vi "GetPos.vi"(0 "Axis In":T1=enum."Y", 11 "error in (no error)":errorcluster) -> (4 "Axis Out":T1=enum."Y", 6 "Position":dbl, 10 "Encoder Counts":i32, 15 "error out":errorcluster)   [LabVIEW 2009]
uses:
  typedefs/AxisSelect_Enum.ctl
  globals/AxisSpace.vi
  typedefs/Ultra3000/Func.ctl
  typedefs/Ultra3000/Cmds.ctl
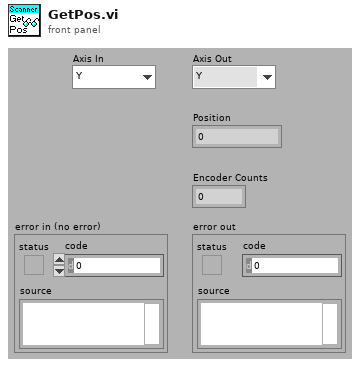
[diagram p1: front panel]
types:
  T1 = typedef "AxisSelect_Enum.ctl" = enum16{"X", "Y", "Z", "Axis Space"}
  T2 = typedef "Cmds.ctl" = u16
  T3 = typedef "Func.ctl" = u16
  T4 = typedef "AxisSpaceCfg.ctl" = T5[]
  T5 = typedef "AxisCfg.ctl" = cluster{"Addr":u8, "Conv Factor":dbl, "Forward Limit":dbl, "Reverse Limit":dbl, "Enable Limits":bool}
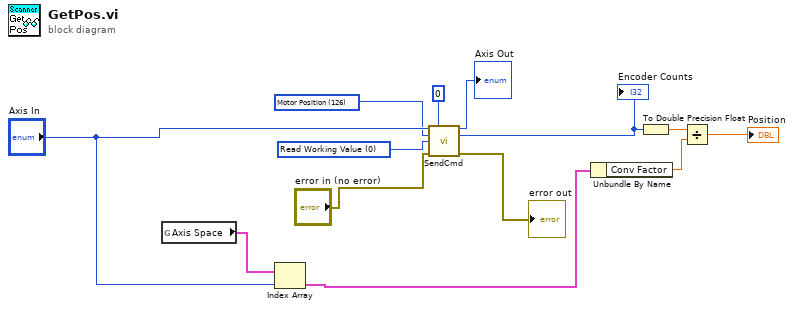
[diagram p0: block diagram]
diagram:
  w7 = T2 126 items=["Motor Position"=126, "Velocity Motor"=133, "Power-Up Status"=1, "Drive Name"=6, "Position Window Size"=22, "Position Window Time"=23, "Zero Speed Limit"=34, "Speed Window Size"=35, "Up to Speed Limit"=37, "Forward Current Limit"=47, "Reverse Current Limit"=48, "Override Mode"=67, "Operation Mode"=90, "Host Control Mode"=97, "Reset Drive"=106, "Drive Enable"=107, "Setpoint Current"=108, "Setpoint Velocity"=109, "Setpoint Acceleration"=110, "Reset Faults"=111, "Position Comparator"=349, "Postition Comparator Polarity"=350, "Position Rollover Enable"=404, "Baud Rate"=80, "Frame Format"=81, "Drive Address"=82, "Broadcast Address"=83, "Auto-start Indexing"=88, "Start Index"=112, "Host Index"=184, "Index Type"=174, "Index Dist/Pos"=175, "Index Reg Dist"=176, "Index Velocity"=177, "Index Acceleration"=178, "Index Deceleration"=179, "Index Dwell"=180, "Index Count"=181, "Index Termination"=182, "Index Pointer"=183, "Index Abort Deceleration"=185, "Positive Soft Pos Limit"=216, "Negative Soft Pos Limit"=217] ("Command")
  w4 = T3 0 items=["Read Working Value", "Write Working Value", "Read Non-Volatile Value", "Write Non-Volatile and Woring Value", "Copy Non-Volatile Value to Working Value", "Copy Working Value to Non-Volatile Value", "Read Default Value", "Copy Default Value to Non-Volatile and Working Values", "Read Min Value", "Read Max Value", "Read Array Index Min", "Read Array Index Max"] ("Function")
  n1 = global read "AxisSpace.vi" "Axis Space"() -> (w9:T4)
  n2 = Index Array(array=w9, index="Axis In") -> (element=w10:T5)
  n3 = call "SendCmd.vi"("Axis In"="Axis In", "Data Length Constant (0)"=u8 0, "Command"=w7, "Function"=w4, "error in (no error)"="error in (no error)") -> ("Axis Out"=→"Axis Out":T1, "Data"=w6:i32, "error out"=→"error out":errorcluster)  [unwired: 7 in, 1 out]
  "Encoder Counts" <- w6
  n4 = Unbundle By Name(w10) -> ("Conv Factor"=w11:dbl)
  n5 = To Double Precision Float(number=w6) -> (double precision float=w12:dbl)
  n6 = Divide(x=w12, y=w11) -> (x/y=→"Position":dbl)
